vi "VSCode-dummy.vi"(9 "Make new code?":bool, 11 "Enter your IP address":string="10.0.0.161") -> (0 "output cluster":errorcluster, 3 "standard output":string="Linux ev3dev 4.14.117-ev3dev-2.3.4-ev3 #1 PREEMPT Thu May 9 15:13:01 CDT 2019 armv5tejl\n             _____     _\n   _____   _|___ /  __| | _____   __\n  / _ \\ \\ / / |_ \\ / _` |/ _ \\ \\ / /\n |  __/\\ V / ___) | (_| |  __/\\ V /\n  \\___| \\_/ |____/ \\__,_|\\___| \\_/\n\nDebian stretch on LEGO MINDSTORMS EV3!\n")   [LabVIEW 2019]
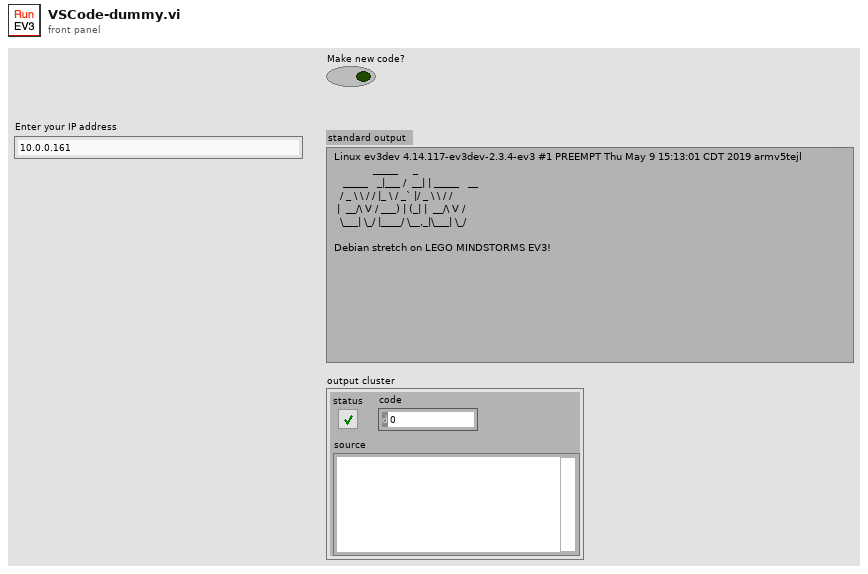
[diagram p1: front panel]
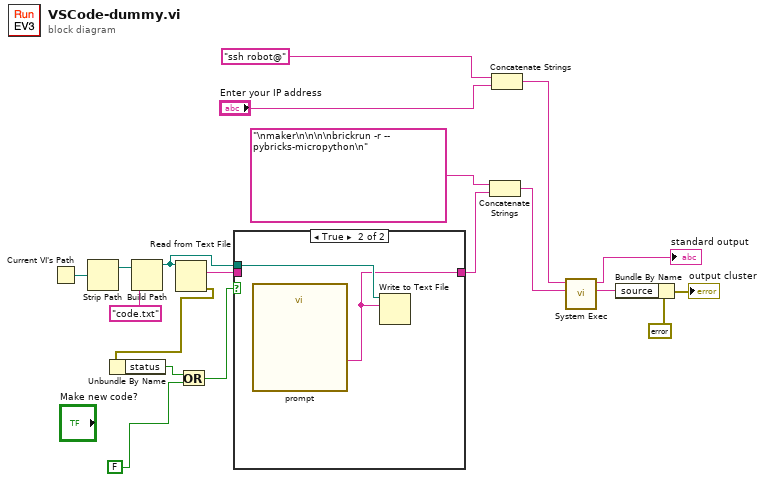
[diagram p0: block diagram]
diagram:
  n1 = Current VI's Path() -> (path=w18:path)
  n2 = Strip Path(path=w18) -> (stripped path=w17:path)  [unwired: 1 out]
  n3 = Build Path(base path=w17, name or relative path="code.txt") -> (appended path=w8:path)
  n4 = Read from Text File(file (use dialog)=w8) -> (text=w9:string, error out=w6:errorcluster)  [unwired: 3 in, 2 out]
  n5 = Unbundle By Name(w6) -> ("status"=w5:bool)
  n6 = Or(x=w5, y=FALSE) -> (x .or. y?=w7:bool)
  n7 = case shown="True" w7 {
    tunnel: w8 -> [_ w22]
    tunnel: [w20 w21] -> w10
    tunnel: w9 -> [w20 _]
    frame False {
    }
    frame True {
      n8 = call "prompt.vi"() -> ("Code"=w21:string)  [unwired: 17 in, 2 out]
      n9 = Write to Text File(file (use dialog)=w22, text=w21) -> ()  [unwired: 2 in, 3 out]
    }
  }
  n10 = Concatenate Strings("\nmaker\n\n\n\nbrickrun -r -- pybricks-micropython\n" ("standard input"), w10) -> (w2:string)
  n11 = Concatenate Strings("ssh robot@" ("command line"), "Enter your IP address") -> (w1:string)
  n12 = call <vilib>:"System Exec.vi"("standard input"=w2, "command line"=w1) -> ("standard error"=w16:string, "standard output"=→"standard output":string)  [unwired: 6 in, 2 out]
  n13 = Bundle By Name(cluster=errorcluster {"status"=FALSE, "code"=0, "source"=""} ("error constant"), "source"=w16) -> (→"output cluster":errorcluster)
